vi "提取系统回应.vi"(11 "字符串":string) -> (3 "系统回应":string)   [LabVIEW 2014]
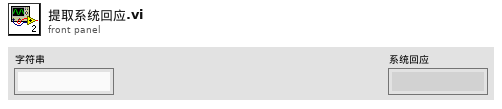
[diagram p1: front panel]
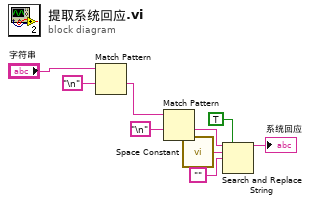
[diagram p0: block diagram]
diagram:
  n1 = Match Pattern(string="字符串", regular expression="\n") -> (after substring=w7:string)  [unwired: 1 in, 3 out]
  n2 = Match Pattern(string=w7, regular expression="\n") -> (after substring=w6:string)  [unwired: 1 in, 3 out]
  n3 = call <vilib>:"Space Constant.vi"() -> ("String"=w5:string)
  n4 = Search and Replace String(replace all?=TRUE ("替换全部？(F)"), input string=w6, search string=w5, replace string="") -> (result string=→"系统回应":string)  [unwired: 4 in, 3 out]
